vi "calculateDAC.vi"(4 "min":dbl[](array[numeric]), 5 "max":dbl[](array[numeric]), 7 "settings":T1, 8 "working":bool[](array[boolean]), 9 "old DAC":dbl[](array[numeric]), 11 "real":dbl[](array[numeric])) -> (0 "new min":dbl[](array[numeric]), 1 "isok":bool, 2 "new DAC":dbl[](array[numeric]), 3 "amplitude":dbl[](array[numeric]), 6 "new max":dbl[](array[numeric]))   [LabVIEW 2012]
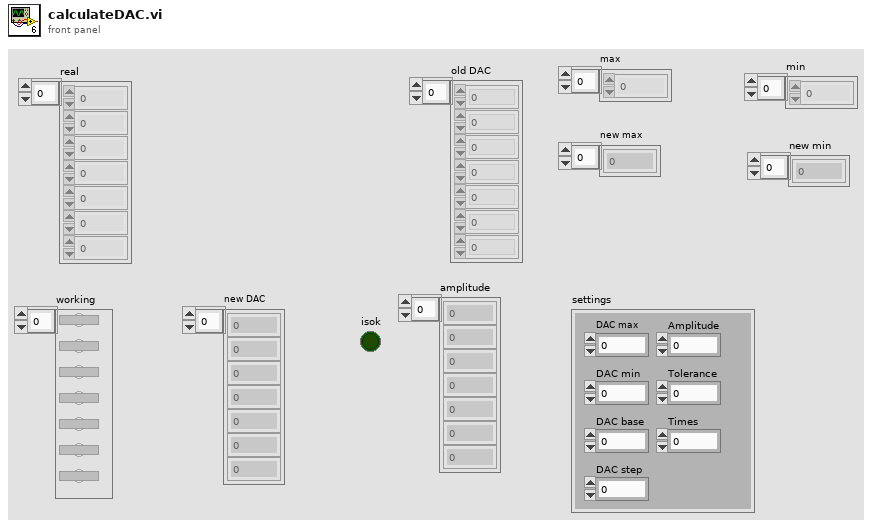
[diagram p1: front panel]
types:
  T1 = cluster{"DAC max":dbl, "DAC min":dbl, "DAC base":dbl, "DAC step":dbl, "Amplitude":dbl, "Tolerance":dbl, "Times":dbl}
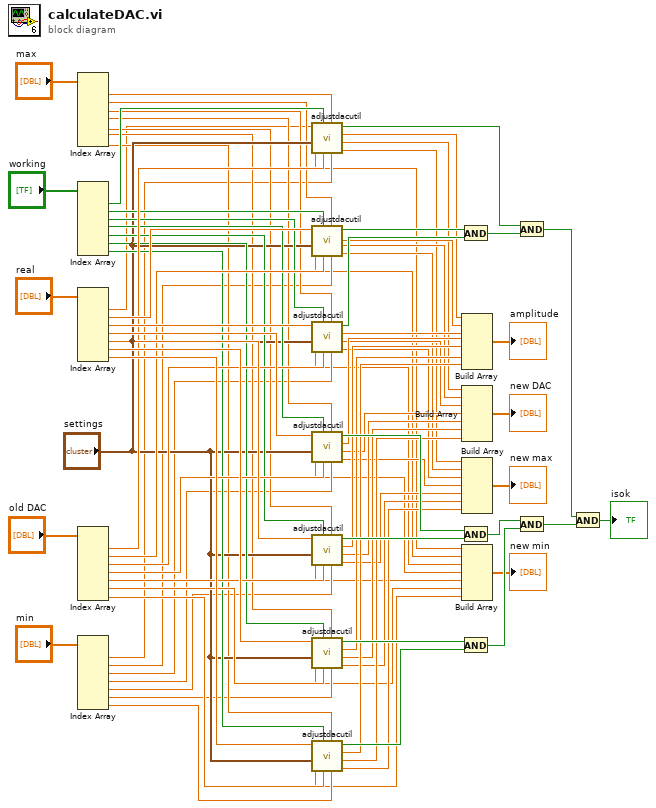
[diagram p0: block diagram]
diagram:
  n1 = Index Array(array="max") -> (element #1=w32:dbl, element #2=w31:dbl, element #3=w30:dbl, element #4=w29:dbl, element #5=w28:dbl, element #6=w27:dbl, element #7=w26:dbl)  [unwired: 7 in]
  n2 = Index Array(array="working") -> (element #1=w63:bool, element #2=w62:bool, element #3=w61:bool, element #4=w60:bool, element #5=w59:bool, element #6=w58:bool, element #7=w57:bool)  [unwired: 7 in]
  n3 = Index Array(array="real") -> (element #1=w1:dbl, element #2=w76:dbl, element #3=w75:dbl, element #4=w74:dbl, element #5=w73:dbl, element #6=w72:dbl, element #7=w71:dbl)  [unwired: 7 in]
  n4 = Index Array(array="old DAC") -> (element #1=w64:dbl, element #2=w65:dbl, element #3=w66:dbl, element #4=w67:dbl, element #5=w68:dbl, element #6=w69:dbl, element #7=w70:dbl)  [unwired: 7 in]
  n5 = Index Array(array="min") -> (element #1=w19:dbl, element #2=w20:dbl, element #3=w21:dbl, element #4=w22:dbl, element #5=w23:dbl, element #6=w24:dbl, element #7=w25:dbl)  [unwired: 7 in]
  n6 = call "adjustdacutil.vi"("min"=w19, "max"=w32, "ori dac"=w64, "work"=w63, "settings"="settings", "real"=w1) -> ("new max"=w17:dbl, "dac"=w42:dbl, "amplitude"=w49:dbl, "ok"=w56:bool, "new min"=w10:dbl)  [unwired: 1 in]
  n7 = call "adjustdacutil.vi"("min"=w20, "max"=w31, "ori dac"=w65, "work"=w62, "settings"="settings", "real"=w76) -> ("new max"=w16:dbl, "dac"=w41:dbl, "amplitude"=w48:dbl, "ok"=w55:bool, "new min"=w9:dbl)  [unwired: 1 in]
  n8 = call "adjustdacutil.vi"("min"=w21, "max"=w30, "ori dac"=w66, "work"=w61, "settings"="settings", "real"=w75) -> ("new max"=w15:dbl, "dac"=w40:dbl, "amplitude"=w47:dbl, "ok"=w54:bool, "new min"=w8:dbl)  [unwired: 1 in]
  n9 = call "adjustdacutil.vi"("min"=w22, "max"=w29, "ori dac"=w67, "work"=w60, "settings"="settings", "real"=w74) -> ("new max"=w14:dbl, "dac"=w39:dbl, "amplitude"=w46:dbl, "ok"=w53:bool, "new min"=w7:dbl)  [unwired: 1 in]
  n10 = call "adjustdacutil.vi"("min"=w23, "max"=w28, "ori dac"=w68, "work"=w59, "settings"="settings", "real"=w73) -> ("new max"=w13:dbl, "dac"=w38:dbl, "amplitude"=w45:dbl, "ok"=w52:bool, "new min"=w6:dbl)  [unwired: 1 in]
  n11 = call "adjustdacutil.vi"("min"=w24, "max"=w27, "ori dac"=w69, "work"=w58, "settings"="settings", "real"=w72) -> ("new max"=w12:dbl, "dac"=w37:dbl, "amplitude"=w44:dbl, "ok"=w51:bool, "new min"=w5:dbl)  [unwired: 1 in]
  n12 = call "adjustdacutil.vi"("min"=w25, "max"=w26, "ori dac"=w70, "work"=w57, "settings"="settings", "real"=w71) -> ("new max"=w11:dbl, "dac"=w36:dbl, "amplitude"=w43:dbl, "ok"=w50:bool, "new min"=w4:dbl)  [unwired: 1 in]
  n13 = And(x=w55, y=w54) -> (x .and. y?=w83:bool)
  n14 = And(x=w53, y=w52) -> (x .and. y?=w82:bool)
  n15 = And(x=w51, y=w50) -> (x .and. y?=w81:bool)
  n16 = Build Array(w49, w48, w47, w46, w45, w44, w43) -> (→"amplitude":dbl[])
  n17 = Build Array(w42, w41, w40, w39, w38, w37, w36) -> (→"new DAC":dbl[])
  n18 = Build Array(w17, w16, w15, w14, w13, w12, w11) -> (→"new max":dbl[])
  n19 = Build Array(w10, w9, w8, w7, w6, w5, w4) -> (→"new min":dbl[])
  n20 = And(x=w56, y=w83) -> (x .and. y?=w80:bool)
  n21 = And(x=w82, y=w81) -> (x .and. y?=w79:bool)
  n22 = And(x=w80, y=w79) -> (x .and. y?=→"isok":bool)
